vi "FlushListenerProcess.vi"(8 "error in (no error)":errorcluster, 10 "process name":string, 11 "Qbus in":refnum<class "Qbus.lvclass">) -> (0 "error in (no error)":errorcluster, 3 "Qbus out":refnum<class "Qbus.lvclass">)   [LabVIEW 2017, in "Qbus.lvclass"]
uses:
  <vilib>/addons/Qbus/Qbus.lvclass
  <vilib>/addons/Qbus/Qbus.lvclass/Qbus.ctl
  <vilib>/addons/Qbus/controls/message.ctl
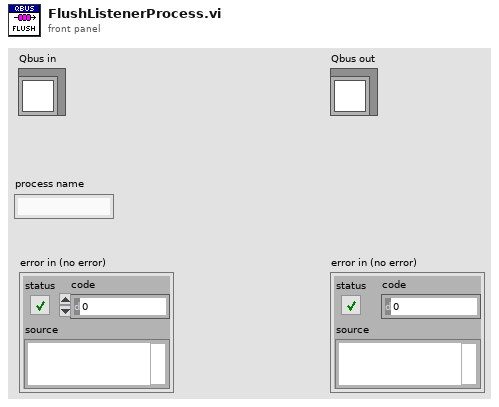
[diagram p1: front panel]
types:
  T1 = typedef "Qbus.lvclass/data.ctl" = cluster{"Queues":variant, "Subscriptions":variant, "MasterQ":string}
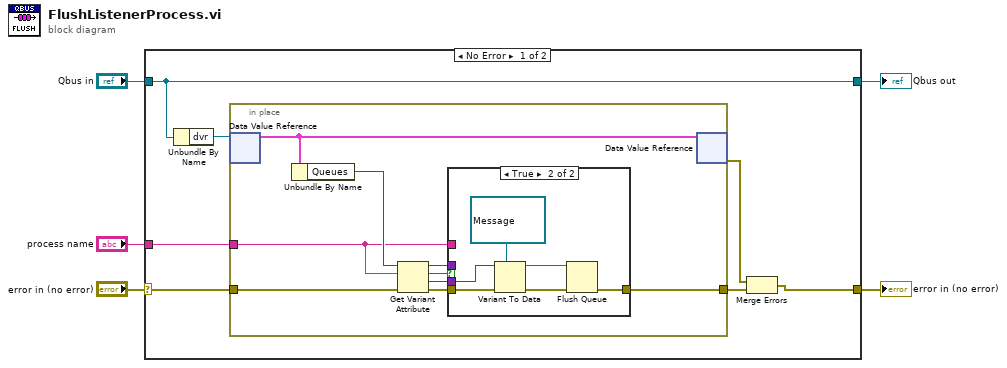
[diagram p0: block diagram]
diagram:
  n1 = case shown="No Error" "error in (no error)" {
    selector: "error in (no error)" -> [w8 w30]
    tunnel: [w7 w30] -> w4
    tunnel: [w12 w29] -> w2
    tunnel: "Qbus in" -> [w12 w29]
    tunnel: "process name" -> [w10 _]
    frame No Error {
      n2 = Unbundle By Name(w12) -> ("dvr"=w11:refnum<data-value>)
      n3 = in-place {
        in-place-border: w8 -> [w21]
        in-place-border: w10 -> [w16]
        in-place-border: [w15] -> w6
        n4 = in-place-dvr #1(w11) -> (w14:T1)  [unwired: 1 out]
        n5 = Unbundle By Name(w14) -> ("Queues"=w18:variant)
        n6 = Get Variant Attribute(Variant=w18, name=w16, error in=w21) -> (duplicate Variant=w17:variant, found=w20:bool, value=w13:variant, error out=w19:errorcluster)  [unwired: 1 in]
        n7 = case shown="True" w20 {
          tunnel: w19 -> [w22 w28]
          tunnel: w17 -> [_ _]
          tunnel: w16 -> [_ _]
          tunnel: [w22 w23] -> w15
          tunnel: w13 -> [_ w27]
          frame False {
          }
          frame True {
            n8 = Variant To Data(error in=w28, type=refnum<queue> refnum ("queue out"), Variant=w27) -> (data=w24:refnum<queue>, error out=w25:errorcluster)
            n9 = Flush Queue(queue=w24, error in (no error)=w25) -> (error out=w23:errorcluster)  [unwired: 2 out]
          }
        }
        n10 = in-place-dvr #1(w14) -> (w9:errorcluster)  [unwired: 1 out]
      }
      n11 = Merge Errors(w9, w6) -> (w7:errorcluster)
    }
    frame Error {
    }
  }
  "error in (no error)" <- w4
  "Qbus out" <- w2
